vi "Nested Alias Unique.vi"(10 "Nested Alias":string, 11 "Ex Queue Actor in":refnum<class "Ex Queue Actor.lvclass">) -> (2 "Nested Alias Unique?":bool)   [LabVIEW 2021, in "Ex Queue Actor.lvlib" / "Ex Queue Actor.lvclass"]
uses:
  Ex Queue Actor.lvclass
  Ex Queue Actor.lvclass/Ex Queue Actor.ctl
  Actor/Queue Actor/Queue Actor.lvclass
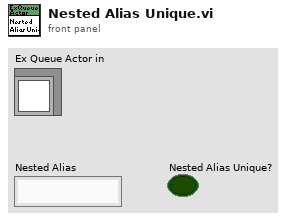
[diagram p1: front panel]
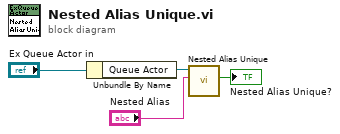
[diagram p0: block diagram]
diagram:
  n1 = Unbundle By Name("Ex Queue Actor in") -> ("Queue Actor"=w3:refnum<class "Queue Actor.lvclass">)
  n2 = call-dynamic "Nested Alias Unique.vi"("Nested Alias"="Nested Alias", "Queue Actor in"=w3) -> ("Nested Alias Unique?"=→"Nested Alias Unique?":bool)  [unwired: 9 in]
